vi "Set Controls(Buttons).vi"(2 "Button Secondary":T1(ring), 3 "Button Primary":T2) -> (0 "Button Secondary":bool, 1 "Button Primary":bool)   [LabVIEW 2014]
uses:
  TypeDefs/Button Actions.ctl
  TypeDefs/SRE Enum.ctl
  Support Code/Robot Global Data.vi
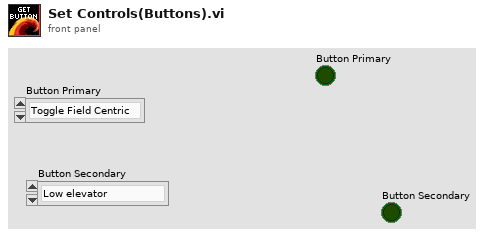
[diagram p1: front panel]
types:
  T1 = enum16{"Low elevator", "High elevator", "Claw up", "Claw Down", "Open/Close claw"}
  T2 = typedef "Button Actions.ctl" = enum16{"Toggle Field Centric", "Gyro Reset", "Clear Faults", "Reduce Speed"}
  T3 = typedef "SRE Enum.ctl" = enum16{"Start", "Run", "End"}
  T4 = enum16{"Left X", "Left Y", "Left trigger", "R trigger", "R X", "R Y"}[]
  T5 = enum16{"X left ", "Y left", "Z left", "X right", "Y right", "Z right"}[]
  T6 = enum16{"Left X", "Left Y", "Left trigger", "R trigger", "R X", "R Y"}
  T7 = enum16{"X left ", "Y left", "Z left", "X right", "Y right", "Z right"}
  T8 = enum16{"A", "B", "X", "Y", "Left bumper", "Right bumper", "Back", "Start", "Left Joystick down", "Right Joystick down"}[]
  T9 = enum16{"Trigger Left", "2 Left", "3 Left", "4 Left", "5 Left", "6 Left", "7 Left", "8 Left", "9 Left", "10 Left", "11 Left", "Trigger Right", "2 Right", "3 Right", "4 Right", "5 Right", "6 Right", "7 Right", "8 Right", "9 Right", "10 Right", "11 Right"}[]
  T10 = enum16{"A", "B", "X", "Y", "Left bumper", "Right bumper", "Back", "Start", "Left Joystick down", "Right Joystick down"}
  T11 = enum16{"Trigger Left", "2 Left", "3 Left", "4 Left", "5 Left", "6 Left", "7 Left", "8 Left", "9 Left", "10 Left", "11 Left", "Trigger Right", "2 Right", "3 Right", "4 Right", "5 Right", "6 Right", "7 Right", "8 Right", "9 Right", "10 Right", "11 Right"}
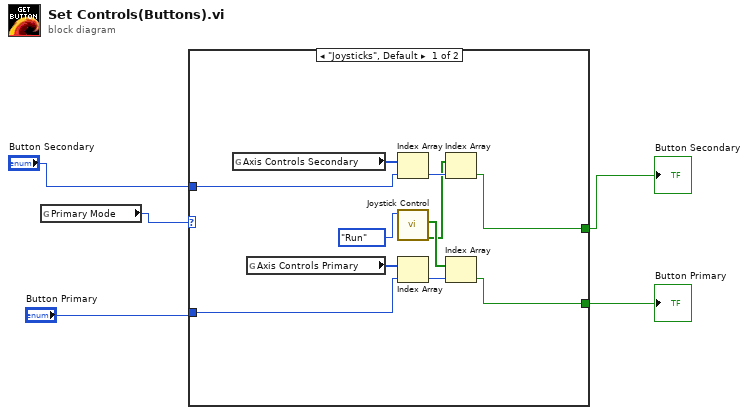
[diagram p0: block diagram]
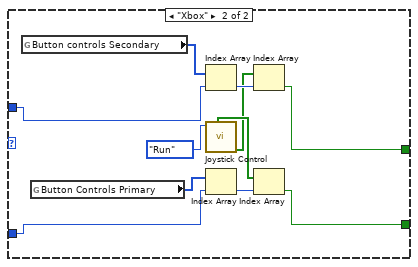
[diagram p2: hidden frame]
diagram:
  n1 = global read "Robot Global Data.vi" "Primary Mode"() -> (w5:enum16{"Joysticks", "Xbox"})
  n2 = case shown="\"Joysticks\", Default" w5 {
    tunnel: "Button Primary" -> [w11 w23]
    tunnel: "Button Secondary" -> [w10 w24]
    tunnel: [w6 w17] -> w1
    tunnel: [w7 w19] -> w2
    frame "Joysticks", Default {
      n3 = global read "Robot Global Data.vi" "Axis Controls Secondary"() -> (w16:T4)
      n4 = global read "Robot Global Data.vi" "Axis Controls Primary"() -> (w12:T5)
      n5 = Index Array(array=w16, index=w10) -> (element=w14:T6)
      n6 = call "Joystick Control.vi"("Enum"=SRE_Enum."Run") -> ("Buttons Output Secondary"=w8:bool[], "Button Output PJ"=w9:bool[])  [unwired: 3 in, 4 out]
      n7 = Index Array(array=w12, index=w11) -> (element=w13:T7)
      n8 = Index Array(array=w8, index=w14) -> (element=w6:bool)
      n9 = Index Array(array=w9, index=w13) -> (element=w7:bool)
    }
    frame "Xbox" {
      n10 = global read "Robot Global Data.vi" "Button controls Secondary"() -> (w21:T8)
      n11 = global read "Robot Global Data.vi" "Button Controls Primary"() -> (w22:T9)
      n12 = Index Array(array=w21, index=w24) -> (element=w26:T10)
      n13 = call "Joystick Control.vi"("Enum"=SRE_Enum."Run") -> ("Buttons Output Secondary"=w18:bool[], "Buttons Output PX"=w20:bool[])  [unwired: 3 in, 4 out]
      n14 = Index Array(array=w22, index=w23) -> (element=w27:T11)
      n15 = Index Array(array=w18, index=w26) -> (element=w17:bool)
      n16 = Index Array(array=w20, index=w27) -> (element=w19:bool)
    }
  }
  "Button Primary" <- w2
  "Button Secondary" <- w1
